vi "Priority.vi"(8 "error in (no error)":errorcluster, 11 "FileExistChecker in":refnum<class "FileExistChecker.lvclass">) -> (0 "error out":errorcluster, 2 "Priority":u16, 3 "FileExistChecker out":refnum<class "FileExistChecker.lvclass">)   [LabVIEW 2020]
uses:
  FileExistChecker.lvclass
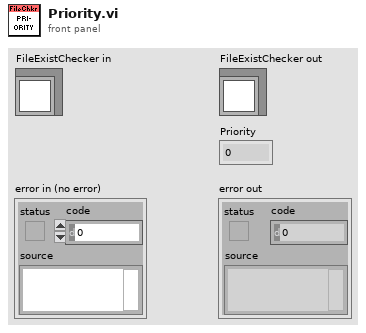
[diagram p1: front panel]
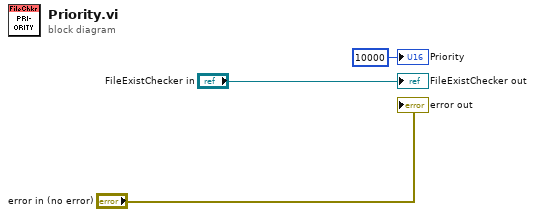
[diagram p0: block diagram]
diagram:
  "error out" <- "error in (no error)"
  "FileExistChecker out" <- "FileExistChecker in"
  "Priority" <- u16 10000 ("Priority")
